vi "rs3 free error.vi"(8 "error in (no error)":errorcluster, 11 "error in":u64) -> (0 "error out 2":errorcluster, 3 "error out":u64)   [LabVIEW 2017, in "libRealSense3.lvlib"]
doc: "void rs_free_error (rs_error * error);"
uses:
  libRealSense3.lvlib
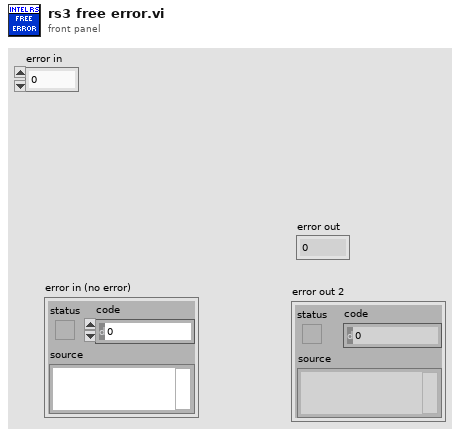
[diagram p1: front panel]
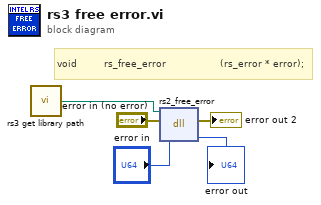
[diagram p0: block diagram]
diagram:
  # "void         rs_free_error                  (rs_error * error);"
  n1 = call "rs3 get library path.vi"() -> ("Realsense 2 Library Path"=w1:path)
  n2 = dll-call lib="C:/Users/agrunnet/Documents/libRealSense6/realsense2.dll" fn="rs2_free_error"(path in=w1, error in="error in (no error)", "error"="error in") -> (error out=→"error out 2":errorcluster, "error"=→"error out":u64)  [unwired: 2 in, 1 out]
